vi "Variable Launch Angle and Speed Trajectory.vi"() -> ()   [LabVIEW 2016]
panel:
  out "Trajectory Graph":cluster{"Y Values":dbl[], "Y Values":dbl[]}(graph)
  out "X Velocity":dbl
  out "Impact Time":dbl
  out "Launch Speed":dbl
  out "Launch Angle":dbl
  out "Target Velocity":dbl
  in  "Impact Angle":dbl(knob) scale=3.141592653589793..-1.5708
  in  "Vertical Distance from Target":dbl(slide) scale=-10.0..10.0
  in  "Horizontal Distance":dbl(slide) scale=0.0..10.0
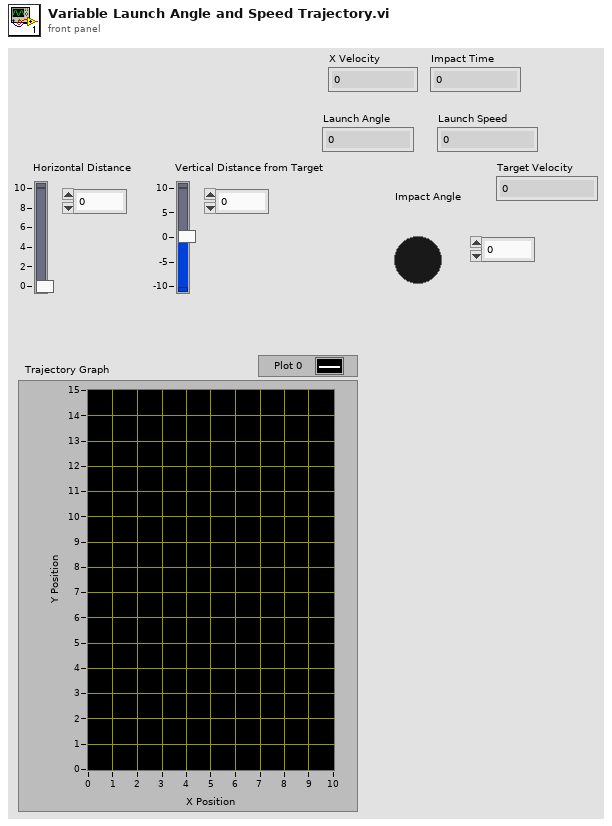
[diagram p1: front panel]
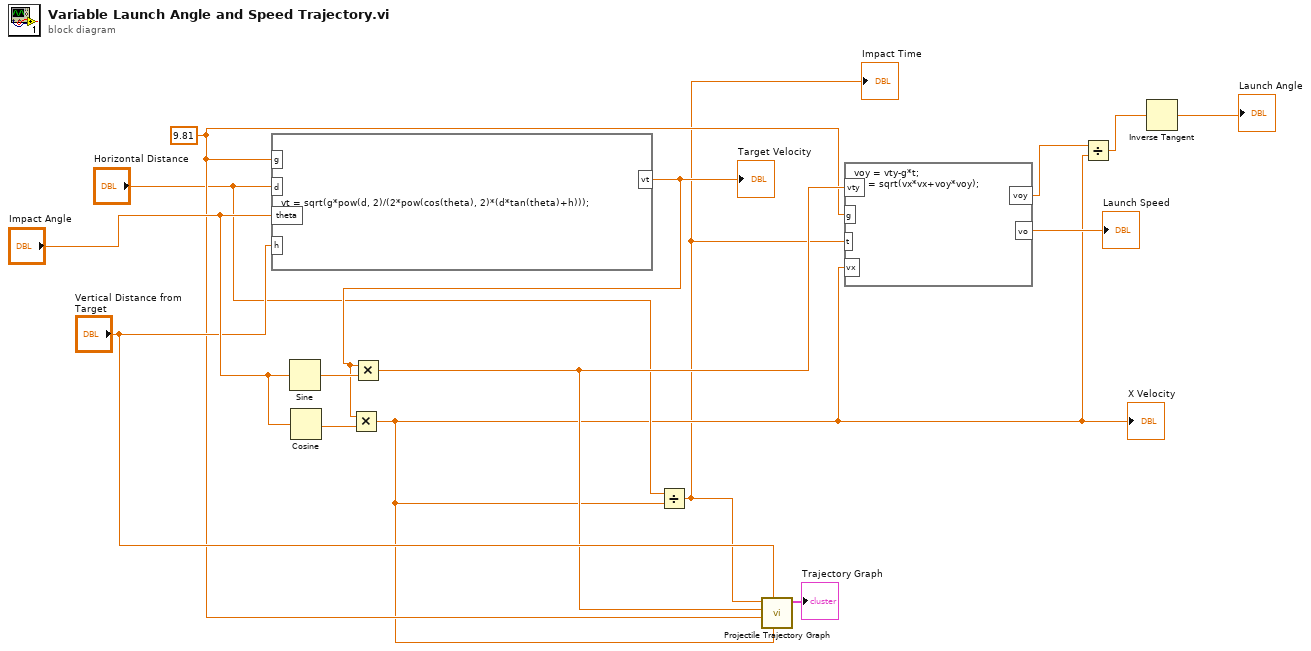
[diagram p0: block diagram]
diagram:
  w9 = 9.81 ("input variable")
  n1 = formula code="vt = sqrt(g*pow(d, 2)/(2*pow(cos(theta), 2)*(d*tan(theta)+h)));"("g"=w9, "d"="Horizontal Distance", "theta"="Impact Angle", "h"="Vertical Distance from Target") -> ("vt"=w12:dbl)
  "Target Velocity" <- w12
  n2 = Sine(x="Impact Angle") -> (sin(x)=w14:dbl)
  n3 = Cosine(x="Impact Angle") -> (cos(x)=w11:dbl)
  n4 = Multiply(x=w12, y=w11) -> (x*y=w3:dbl)
  "X Velocity" <- w3
  n5 = Multiply(x=w12, y=w14) -> (x*y=w10:dbl)
  n6 = Divide(x="Horizontal Distance", y=w3) -> (x/y=w2:dbl)
  "Impact Time" <- w2
  n7 = call "Projectile Trajectory Graph.vi"("X Velocity"=w3, "Initial Height"="Vertical Distance from Target", "Gravitational Acceleration"=w9, "Initial Y Velocity"=w10, "End Time"=w2) -> ("Trajectory Graph"=→"Trajectory Graph":cluster{"Y Values":dbl[], "Y Values":dbl[]})  [unwired: 6 in]
  n8 = formula code="voy = vty-g*t;\nvo = sqrt(vx*vx+voy*voy);"("vty"=w10, "t"=w2, "g"=w9, "vx"=w3) -> ("voy"=w6:dbl, "vo"=→"Launch Speed":dbl)
  n9 = Divide(x=w6, y=w3) -> (x/y=w5:dbl)
  n10 = Inverse Tangent(1:w5) -> (0:→"Launch Angle":dbl)
